vi "X682 Camera Calibration Tester Program Ver1.0.0.0.vi"() -> ()   [LabVIEW 2017]
uses:
  Thorlabs.MotionControl.Controls.dll
  Ctrls/MainStep.ctl
  Ctrls/AllControls.ctl
  <vilib>/Utility/miscctls.llb/LVRowAndColumnTypeDef.ctl
  ComVIS/Files/Ini/WriteIniFiles_ByVarient.vi
  Thorlabs.MotionControl.IntegratedStepperMotorsCLI.dll
panel:
  in  "LongTravelStageControl":refnum<k24>(container)
  in  "Recipe":string(combo)
  in  "MES Status":bool
  in  "maintenance":bool
  in  "mode":enum32{"Production mode", "Engineering mode"}(tab)
  out "Fail resume":bool caption="TotalResult"
  out "Table":string[][](table)
  out "LogInfo":string caption="Log"
  in  "AlarmData":i32(listbox)=-1
  out "Device state":bool caption="TotalResult"
  out "CT":dbl format="%#_3f"
  in  "ProductID:":string
  in  "TestInfo":T1 {"Yield" format="%#_g%"}
  out "MES_Status":string
  out "TestMode":string
  in  "Stop":bool
  in  "Start":bool
  in  "Exit":bool
  in  "Login":bool
  out "Login_status":string="Operator:Operator"
  out "OpenStatus":string
  in  "error in (no error)":errorcluster caption="错误输入（无错误）"
  # "Dyson X682 Camera Calibration Tester"
  # "Waiting Barcode scanning"
types:
  T1 = cluster{"Total":i32, "OK":i32, "NG":i32, "Yield":dbl}
  T2 = typedef "MainStep.ctl" = enum16{"Initialize", "ReadAllFiles", "ResetHardware", "Run", "Exit"}
  T3 = typedef "AllControls.ctl" = cluster{"MainVI":refnum<vi>, "AlarmInfo":refnum<vi>, "Log":refnum<vi>, "Current CT":refnum<vi>, "ProductID":refnum<vi>, "Device state":refnum<vi>, "MES":refnum<vi>, "mode":refnum<vi>, "TestInfo":refnum<vi>, "SubPnl":refnum<vi>, "Table":refnum<vi>, "MES bool":refnum<vi>, "TestMode":refnum<vi>, "Recipe":refnum<vi>, "Fail resume":refnum<vi>, "LogIn":refnum<vi>, "Start":refnum<vi>, "Maintenance":refnum<vi>, "Stop":refnum<vi>, "Exit":refnum<vi>}
  T4 = enum32{"Invalid", "Standard", "Closed", "Hidden", "Minimized", "Maximized"}
  T5 = enum16{"Ini", "Standby", "Running", "Engineering"}
  T6 = typedef "LVRowAndColumnTypeDef.ctl" = cluster{"Row":i32, "Column":i32}
  T7 = enum32{"invalid app kind", "Development System", "Run Time System", "Student Edition", "Embedded LabVIEW", "Evaluation", "Custom"}
  T8 = typedef "amc_Message Queue.ctl" = refnum<queue>
  T9 = typedef "HD Config.ctl" = cluster{" PC":cluster{"PC Address":u8[], "PC Port":i32}, "FCO":cluster{"COM":refnum<visa-resource-name>, "Baudrate":u32}, "DC Power ":cluster{"COM":refnum<visa-resource-name>, "Baudrate":u32}, "PW3336":cluster{"COM":refnum<visa-resource-name>, "Baudrate":u32}, "Lefoo":cluster{"COM":refnum<visa-resource-name>, "Baudrate":u32}, "Tempt&Hum":cluster{"COM":refnum<visa-resource-name>, "Baudrate":u32}, "DIPC":cluster{"COM":refnum<visa-resource-name>}, "Daemon":cluster{"IP Address":string, "Port":u16, "Retry":u16}, "NFC_Cmd":cluster{"COM":refnum<visa-resource-name>, "Baudrate":u32}, "Fail_resume_mode":bool, "GRR":bool, "NFC _Serial":cluster{"COM":refnum<visa-resource-name>, "Baudrate":u32}}
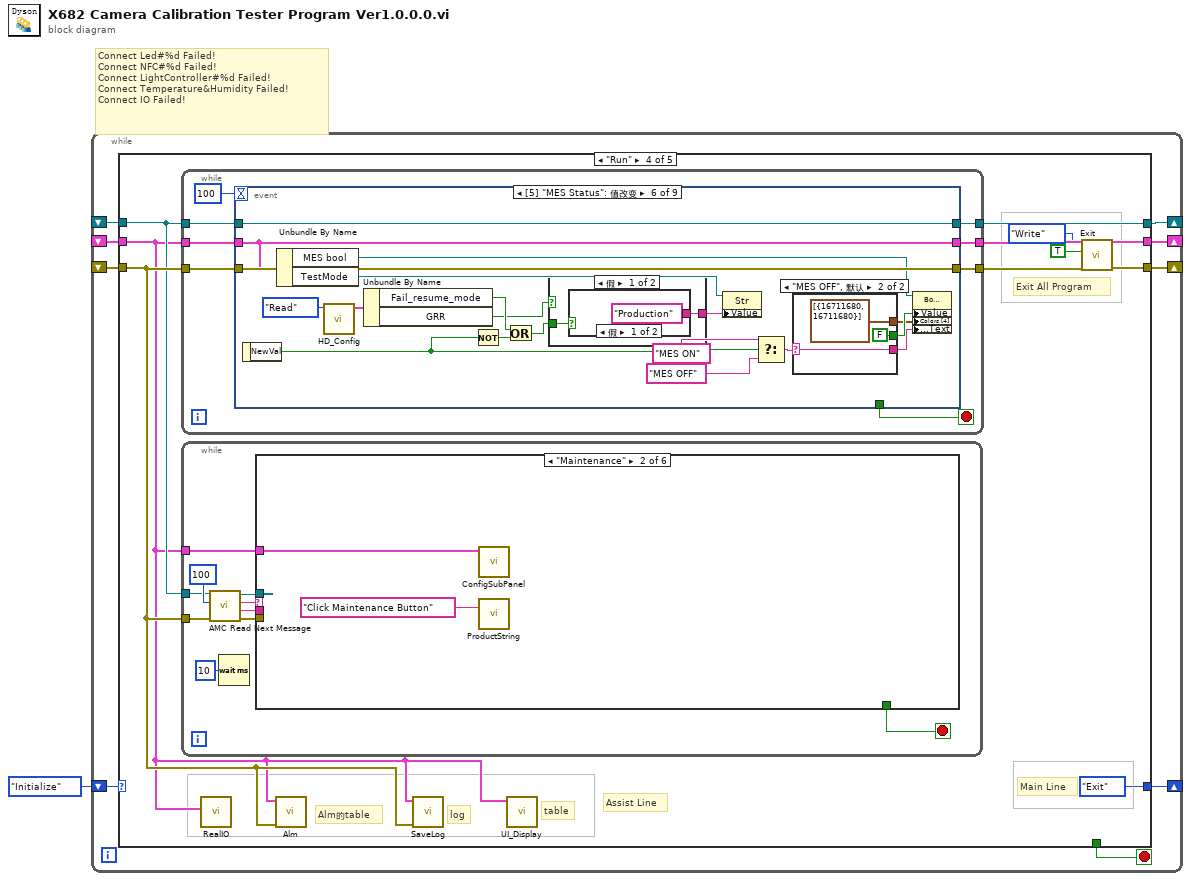
[diagram p0: block diagram]
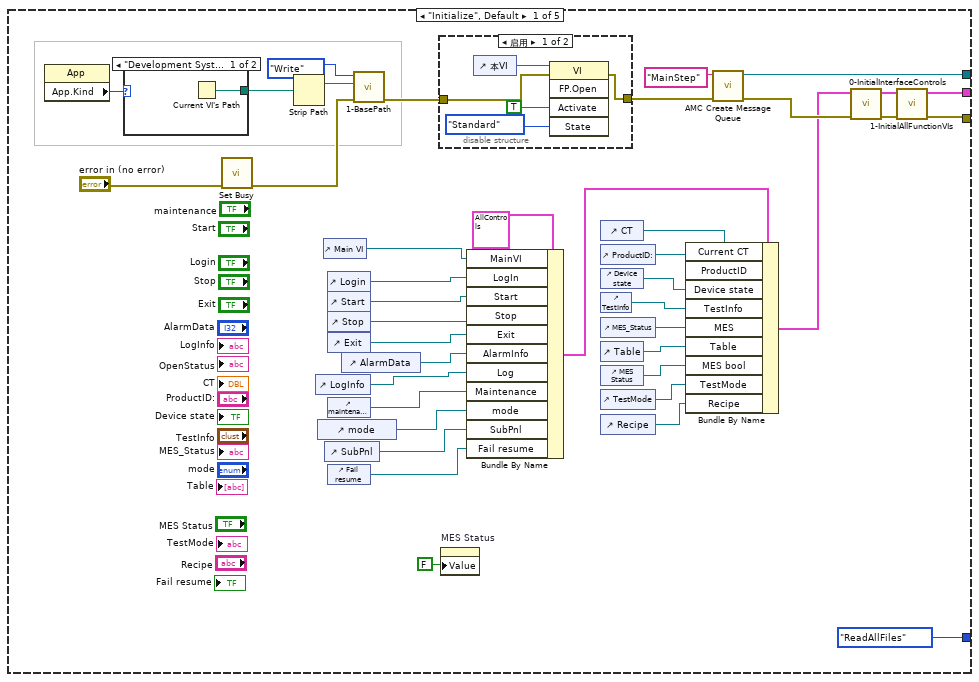
[diagram p2: hidden frame]
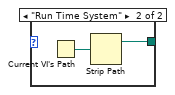
[diagram p4: hidden frame]
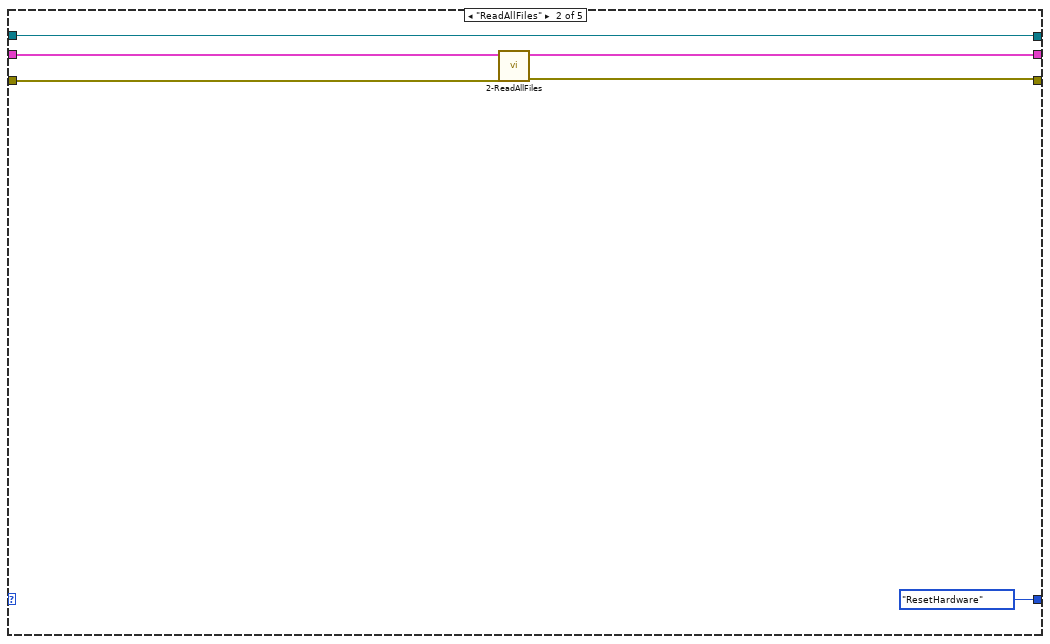
[diagram p5: hidden frame]
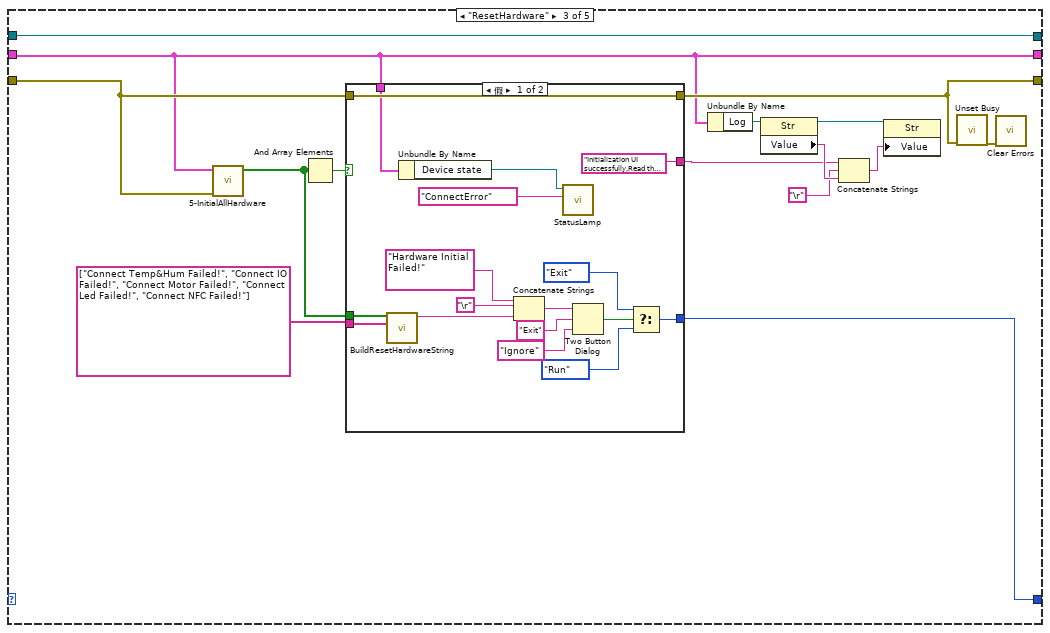
[diagram p6: hidden frame]
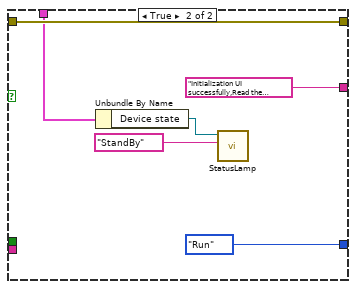
[diagram p7: hidden frame]
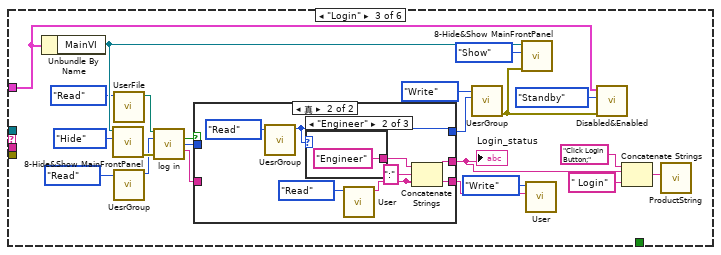
[diagram p9: hidden frame]
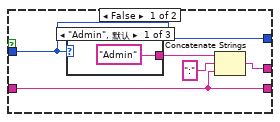
[diagram p10: hidden frame]
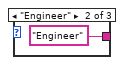
[diagram p11: hidden frame]
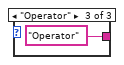
[diagram p12: hidden frame]
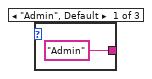
[diagram p13: hidden frame]
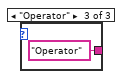
[diagram p14: hidden frame]
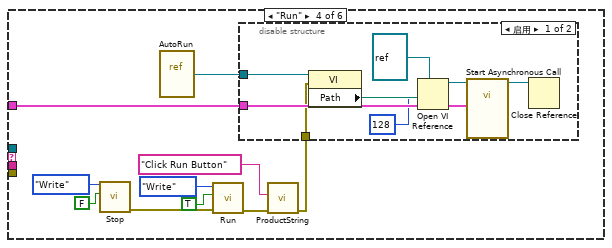
[diagram p15: hidden frame]
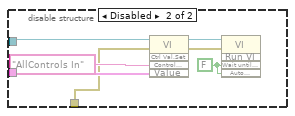
[diagram p16: hidden frame]
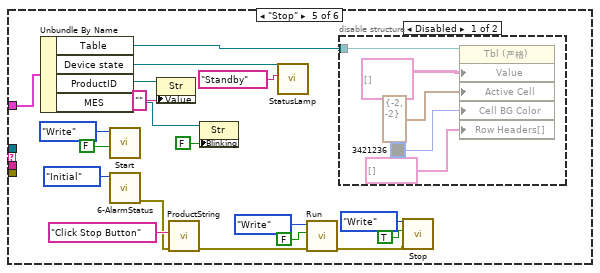
[diagram p17: hidden frame]
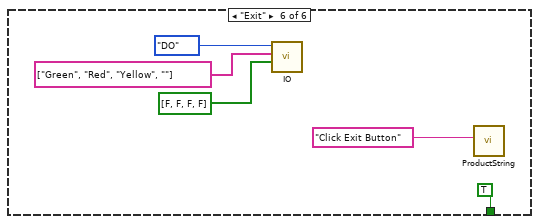
[diagram p19: hidden frame]
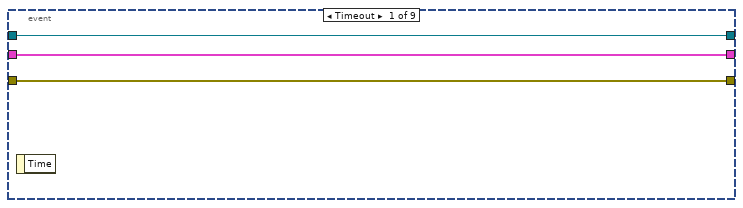
[diagram p20: hidden frame]
diagram:
  # "Connect Led#%d Failed!\nConnect NFC#%d Failed!\nConnect LightController#%d Failed!\nConnect Temperature&Humidity Failed!\nConnect IO Failed!"
  n1 = while {
    shift-right: [w9] -> _
    shift-left: MainStep."Initialize" -> [w10]
    shift-right: [w7] -> _
    shift-left: _ -> [w2]
    shift-right: [w5] -> _
    shift-left: _ -> [w3]
    shift-right: [w6] -> _
    shift-left: _ -> [w4]
    stop <- w8 stop-if-true
    n2 = case shown="\"Run\"" w10 {
      tunnel: [MainStep."ReadAllFiles" MainStep."ResetHardware" w80 MainStep."Exit" MainStep."Exit"] -> w9
      tunnel: [_ _ _ _ TRUE] -> w8
      tunnel: [w37 w60 w76 w107 w347] -> w7
      tunnel: [w45 w64 w79 w112 _] -> w6
      tunnel: [w38 w62 w74 w111 w345] -> w5
      tunnel: w4 -> [_ w64 w79 w105 w348]
      tunnel: w3 -> [_ w63 w74 w104 w345]
      tunnel: w2 -> [_ w61 w77 w106 w346]
      frame "Initialize", Default {
        n3 = property class="App"() -> ("App.Kind"=w49:T7)  [unwired: 2 in, 2 out]
        n4 = case shown="\"Development System\", 默认" w49 {
          tunnel: [w57 w58] -> w48
          frame "Development System", Default {
            n5 = Current VI's Path() -> (path=w57:path)
          }
          frame "Run Time System" {
            n6 = Current VI's Path() -> (path=w59:path)
            n7 = Strip Path(path=w59) -> (stripped path=w58:path)  [unwired: 1 out]
          }
        }
        n8 = call <vilib>:"Set Busy.vi"("error in (no error)"="error in (no error)") -> ("error out"=w17:errorcluster)  [unwired: 9 in, 1 out]
        n9 = Strip Path(path=w48) -> (stripped path=w18:path)  [unwired: 1 out]
        n10 = control-ref of="LogInfo"() -> (w42:refnum<vi>)
        n11 = control-ref of="mode"() -> (w24:refnum<vi>)
        n12 = control-ref of="Main VI"() -> (w35:refnum<vi>)
        n13 = control-ref of="SubPnl"() -> (w22:refnum<vi>)
        n14 = control-ref of="Login"() -> (w25:refnum<vi>)
        n15 = control-ref of="Start"() -> (w26:refnum<vi>)
        n16 = control-ref of="Stop"() -> (w27:refnum<vi>)
        n17 = control-ref of="Exit"() -> (w28:refnum<vi>)
        n18 = control-ref of="maintenance"() -> (w23:refnum<vi>)
        n19 = control-ref of="Fail resume"() -> (w12:refnum<vi>)
        n20 = control-ref of="AlarmData"() -> (w43:refnum<vi>)
        n21 = call "1-BasePath.vi"("error in (no error)"=w17, "Path In"=w18, "Step"=enum16{"Initial", "Write", "Read"}."Write") -> ("error out"=w16:errorcluster)  [unwired: 7 in, 1 out]
        n22 = disable-structure shown="启用" {
          disable-tunnel: w16 -> [w53 w56]
          disable-tunnel: [w51 w56] -> w46
          frame Enabled {
            n23 = control-ref of="本VI"() -> (w55:refnum<vi>)
            n24 = invoke class="VI" method="FP.Open"(reference=w55, error in=w53, "Activate"=TRUE ("激活？"), "State"=T4."Standard" ("状态")) -> (error out=w51:errorcluster)  [unwired: 1 in, 4 out]
          }
          frame Disabled {
          }
        }
        n25 = property on="MES Status" class="Bool (严格)"("Value"=FALSE ("MES Status")) -> ()  [unwired: 2 in, 2 out]
        n26 = Bundle By Name(cluster=T3 {"MainVI"=refnum, "AlarmInfo"=refnum, "Log"=refnum, "Current CT"=refnum, "ProductID"=refnum, "Device state"=refnum, "MES"=refnum, "mode"=refnum, "TestInfo"=refnum, "SubPnl"=refnum, "Table"=refnum, "MES bool"=refnum, "TestMode"=refnum, "Recipe"=refnum, "Fail resume"=refnum, "LogIn"=refnum, "Start"=refnum, "Maintenance"=refnum, "Stop"=refnum, "Exit"=refnum}, "MainVI"=w35, "LogIn"=w25, "Start"=w26, "Stop"=w27, "Exit"=w28, "AlarmInfo"=w43, "Log"=w42, "Maintenance"=w23, "mode"=w24, "SubPnl"=w22, "Fail resume"=w12) -> (w34:T3)
        n27 = control-ref of="CT"() -> (w31:refnum<vi>)
        n28 = control-ref of="ProductID:"() -> (w32:refnum<vi>)
        n29 = control-ref of="Device state"() -> (w33:refnum<vi>)
        n30 = control-ref of="TestInfo"() -> (w30:refnum<vi>)
        n31 = control-ref of="MES_Status"() -> (w29:refnum<vi>)
        n32 = control-ref of="Table"() -> (w20:refnum<vi>)
        n33 = control-ref of="MES Status"() -> (w15:refnum<vi>)
        n34 = control-ref of="TestMode"() -> (w14:refnum<vi>)
        n35 = control-ref of="Recipe"() -> (w13:refnum<vi>)
        n36 = Bundle By Name(cluster=w34, "Current CT"=w31, "ProductID"=w32, "Device state"=w33, "TestInfo"=w30, "MES"=w29, "Table"=w20, "MES bool"=w15, "TestMode"=w14, "Recipe"=w13) -> (w21:T3)
        n37 = call "AMC Create Message Queue.vi"("error in (no error)"=w46, "Message Queue Name"="MainStep" ("Message queue name (unnamed)")) -> ("error out"=w41:errorcluster, "Message Queue out"=w45:T8)  [unwired: 3 in, 5 out]
        n38 = call "0-InitialInterfaceControls.vi"("error in (no error)"=w41, "AllControls IN"=w21) -> ("error out"=w40:errorcluster, "AllControls Out"=w39:T3)  [unwired: 8 in]
        n39 = call "1-InitialAllFunctionVIs.vi"("error in (no error)"=w40, "AllControls IN"=w39) -> ("error out"=w37:errorcluster, "AllControls Out"=w38:T3)  [unwired: 8 in]
      }
      frame "ReadAllFiles" {
        n40 = call "2-ReadAllFiles.vi"("error in (no error)"=w61, "AllControls IN"=w63) -> ("error out"=w60:errorcluster, "AllControls Out"=w62:T3)  [unwired: 8 in]
      }
      frame "ResetHardware" {
        n41 = call "5-InitialAllHardware.vi"("error in (no error)"=w77, "AllControls IN"=w74) -> ("InitalResult"=w78:bool[])  [unwired: 9 in]
        n42 = And Array Elements(Boolean array=w78) -> (logical AND=w66:bool)
        n43 = case shown="假" w66 {
          tunnel: [w88 MainStep."Run"] -> w80
          tunnel: w77 -> [w97 w102]
          tunnel: string[] ["Connect Temp&Hum Failed!", "Connect IO Failed!", "Connect Motor Failed!", "Connect Led Failed!", "Connect NFC Failed!"] -> [w86 _]
          tunnel: w78 -> [w87 _]
          tunnel: [w97 w102] -> w76
          tunnel: ["Initialization UI successfully,Read the configuration parameter successfully,Initialize hardware failure" ("值") "Initialization UI successfully,Read the configuration parameter successfully,Initialize hardware successfully" ("值")] -> w70
          tunnel: w74 -> [w81 w100]
          frame False {
            n44 = call "BuildResetHardwareString.vi"("String"=w86, "Error"=w87) -> ("DataOut"=w85:string)  [unwired: 9 in]
            n45 = Unbundle By Name(w81) -> ("Device state"=w82:refnum<vi>)
            n46 = Concatenate Strings("Hardware Initial Failed!" ("caption"), "\r", w85) -> (w95:string)
            n47 = call "StatusLamp.vi"("State"="ConnectError", "Boolean输入"=w82) -> ()  [unwired: 9 in, 1 out]
            n48 = Two Button Dialog(message=w95, 1:"Ignore" ("F按钮名称（“取消”）"), 2:"Exit" ("T按钮名称（“确定”）")) -> (T button?=w91:bool)
            n49 = Select(t=MainStep."Exit", s=w91, f=MainStep."Run") -> (s? t:f=w88:T2)
          }
          frame True {
            n50 = Unbundle By Name(w100) -> ("Device state"=w98:refnum<vi>)
            n51 = call "StatusLamp.vi"("State"="StandBy", "Boolean输入"=w98) -> ()  [unwired: 9 in, 1 out]
          }
        }
        n52 = Unbundle By Name(w74) -> ("Log"=w71:refnum<vi>)
        n53 = property class="Str"(reference=w71) -> (reference out=w69:refnum<vi>, "Value"=w73:string)  [unwired: 1 in, 1 out]
        n54 = Concatenate Strings(w70, "\r", w73) -> (w68:string)
        n55 = property class="Str"(reference=w69, "Value"=w68) -> ()  [unwired: 1 in, 2 out]
        n56 = call <vilib>:"Unset Busy.vi"("error in (no error)"=w76) -> ("error out"=w75:errorcluster)  [unwired: 10 in]
        n57 = call <vilib>:"Clear Errors.vi"("error in (no error)"=w75) -> ()  [unwired: 5 in, 2 out]
      }
      frame "Run" {
        # "Alm的table"
        # "log"
        # "table"
        # "Exit All Program"
        # "Assist Line"
        # "Main Line"
        n58 = while {
          tunnel: w105 -> [w227]
          tunnel: w104 -> [w226]
          tunnel: w106 -> [w225]
          tunnel: [w224] -> w112
          tunnel: [w223] -> w111
          tunnel: [w222] -> w108
          stop <- w221 stop-if-true
          n59 = event shown="[5] \"MES Status\": 值改变" {
            selector: _ -> [_ _ _ _ _ _ _ _ _]
            dyn-events: _ -> [_ _ _ _ _ _ _ _ _]
            timeout: 100 -> [_ _ _ _ _ _ _ _ _]
            tunnel: w227 -> [w230 w238 w263 w269 w281 w306 w320 w329 w336]
            tunnel: w226 -> [w229 w233 w261 w268 w279 w304 w318 w331 w341]
            tunnel: w225 -> [w228 w237 w262 w271 w280 w305 w319 w328 w337]
            tunnel: [w230 w238 w263 w269 w281 w306 w320 w329 w336] -> w224
            tunnel: [w229 w233 w261 w268 w279 w304 w318 w331 w341] -> w223
            tunnel: [w228 w237 w262 w271 w280 w305 w319 w328 w337] -> w222
            tunnel: [_ _ _ _ _ _ _ w327 w340] -> w221
            event Timeout {
              n60 = event-data() -> ()  [unwired: 1 in, 1 out]
            }
            event "Recipe": Value Change {
              n61 = event-data() -> ("OldVal"=w236:string, "NewVal"=w234:string)  [unwired: 1 in]
              n62 = Not Equal?(x=w236, y=w234) -> (x != y?=w235:bool)
              n63 = call "Run.vi"("Step"=enum16{"Initial", "Write", "Read"}."Read") -> ("Run Out"=w231:bool)  [unwired: 9 in, 1 out]
              n64 = case shown="假" w231 {
                tunnel: w235 -> [w241 _]
                tunnel: w234 -> [w240 _]
                tunnel: w233 -> [w239 _]
                frame False {
                  n65 = case shown="真" w241 {
                    tunnel: w240 -> [_ w255]
                    tunnel: w239 -> [_ w243]
                    frame False {
                    }
                    frame True {
                      w256 = cluster{"Recipe":string} {"Recipe"=""}  # Recipe
                      n66 = call "1-BasePath.vi"("Step"=enum16{"Initial", "Write", "Read"}."Read") -> ("Path Out"=w257:path)  [unwired: 9 in, 1 out]
                      n67 = call "ReadConfigandSetting.vi"("Recipe"=w255, "Path Out"=w257) -> ("TableData"=w244:string[][])  [unwired: 7 in, 2 out]
                      n68 = Bundle By Name(cluster=w256, "Recipe"=w255) -> (w254:cluster{"Recipe":string})
                      n69 = Build Path(base path=w257, name or relative path="data\\Recipe.ini") -> (appended path=w259:path)
                      n70 = Unbundle By Name(w243) -> ("Table"=w242:refnum<vi>)
                      n71 = call-poly "Read&WriteFile.vi"("Variant"=w254, "path"=w259) -> ()  [unwired: 9 in, 1 out]
                      n72 = Delete From Array(array=w244, length=1 ("长度"), index (row)=0 ("索引 (行)")) -> (deleted portion=w252:string[][], array with subset deleted=w250:string[][])  [unwired: 1 in]
                      n73 = call "Select_UUT_Table.vi"("all Title"=w252, "all Table"=w250) -> ("Title"=w251:string[], "Table"=w253:string[][])  [unwired: 8 in]
                      n74 = property class="Tbl (严格)"(reference=w242, "Value"=w253, "Column Headers[]"=w251, "Active Cell"=T6 {"Row"=-2, "Column"=-2} ("活动单元格:活动单元格"), "Cell BG Color"=u32 3421236, "Row Headers[]"=string[] [] ("Row Header Strings[]")) -> ()  [unwired: 1 in, 2 out]
                    }
                  }
                }
                frame True {
                }
              }
            }
            event "Login": Value Change {
              n75 = event-data() -> ("NewVal"=w264:bool)  [unwired: 1 in]
              n76 = case shown="真" w264 {
                tunnel: w263 -> [w267 _]
                tunnel: w262 -> [w266 _]
                frame True {
                  n77 = call "AMC Send Local Message.vi"("error in (no error)"=w266, "Message Name"="Login", "Message Queue in"=w267) -> ()  [unwired: 7 in, 2 out]
                }
                frame False {
                }
              }
            }
            event "maintenance": Value Change {
              n78 = event-data() -> ("NewVal"=w272:bool)  [unwired: 1 in]
              n79 = Unbundle By Name(w268) -> ("mode"=w270:refnum<vi>)
              n80 = case shown="真" w272 {
                tunnel: w270 -> [w278 _]
                tunnel: w269 -> [w275 _]
                tunnel: w268 -> [w274 _]
                frame True {
                  n81 = call "AMC Send Local Message.vi"("Message Name"="Maintenance", "Message Queue in"=w275) -> ()  [unwired: 8 in, 2 out]
                  n82 = property class="TabCtl (严格)"(reference=w278, "Value"=enum32{"Production mode", "Engineering mode"}."Engineering mode" ("值")) -> ()  [unwired: 1 in, 2 out]
                  n83 = call "Disabled&Enabled.vi"("Mode in"=T5."Engineering", "AllControls In"=w274) -> ()  [unwired: 9 in, 1 out]
                }
                frame False {
                }
              }
            }
            event "Start": Value Change {
              n84 = event-data() -> ("NewVal"=w282:bool)  [unwired: 1 in]
              n85 = case shown="真" w282 {
                tunnel: w281 -> [w287 _]
                tunnel: w280 -> [w286 _]
                tunnel: w279 -> [w283 _]
                frame True {
                  n86 = call "AMC Send Local Message.vi"("error in (no error)"=w286, "Message Name"="Run", "Message Queue in"=w287) -> ()  [unwired: 7 in, 2 out]
                  n87 = call "Disabled&Enabled.vi"("Mode in"=T5."Running", "AllControls In"=w283) -> ()  [unwired: 9 in, 1 out]
                }
                frame False {
                }
              }
            }
            event "MES Status": Value Change {
              n88 = event-data() -> ("NewVal"=w289:bool)  [unwired: 1 in]
              n89 = Unbundle By Name(w304) -> ("MES bool"=w297:refnum<vi>, "TestMode"=w288:refnum<vi>)
              n90 = call "HD_Config.vi"("Step"=enum16{"Initial", "Write", "Read"}."Read") -> ("HD Config out"=w296:T9)  [unwired: 9 in, 1 out]
              n91 = Unbundle By Name(w296) -> ("Fail_resume_mode"=w293:bool, "GRR"=w291:bool)
              n92 = Not(x=w289) -> (.not. x?=w295:bool)
              n93 = Or(x=w293, y=w295) -> (x .or. y?=w294:bool)
              n94 = case shown="假" w291 {
                tunnel: w294 -> [w308 _]
                tunnel: [w307 "GRR"] -> w292
                frame False {
                  n95 = case shown="假" w308 {
                    tunnel: ["Production" "Engineering"] -> w307
                    frame False {
                    }
                    frame True {
                    }
                  }
                }
                frame True {
                }
              }
              n96 = property class="Str"(reference=w288, "Value"=w292) -> ()  [unwired: 1 in, 2 out]
              n97 = Select(t="MES ON", s=w289, f="MES OFF") -> (s? t:f=w298:string)
              n98 = case shown="\"MES OFF\", 默认" w298 {
                selector: w298 -> [w312 w315]
                tunnel: [TRUE FALSE] -> w300
                tunnel: [w312 w315] -> w301
                tunnel: [cluster{u32, u32}[] [{6618880, 6618880}] cluster{u32, u32}[] [{16711680, 16711680}]] -> w299
                frame "MES ON" {
                }
                frame "MES OFF", Default {
                }
              }
              n99 = property on="属性节点" class="Bool (严格)"(reference=w297, "Value"=w300, "Colors [4]"=w299, "BoolText.Text"=w301) -> ()  [unwired: 1 in, 2 out]
            }
            event "Stop": Value Change {
              n100 = event-data() -> ("NewVal"=w321:bool)  [unwired: 1 in]
              n101 = case shown="真" w321 {
                tunnel: w320 -> [w326 _]
                tunnel: w319 -> [w325 _]
                tunnel: w318 -> [w322 _]
                frame True {
                  n102 = call "AMC Send Local Message.vi"("error in (no error)"=w325, "Message Name"="Stop", "Message Queue in"=w326) -> ()  [unwired: 7 in, 2 out]
                  n103 = call "Disabled&Enabled.vi"("Mode in"=T5."Standby", "AllControls In"=w322) -> ()  [unwired: 9 in, 1 out]
                }
                frame False {
                }
              }
            }
            event "Exit": Value Change {
              n104 = event-data() -> ("NewVal"=w330:bool)  [unwired: 1 in]
              n105 = case shown="真" w330 {
                tunnel: w329 -> [_ w335]
                tunnel: w328 -> [_ w334]
                tunnel: [_ TRUE] -> w327
                frame False {
                }
                frame True {
                  n106 = call "AMC Send Local Message.vi"("error in (no error)"=w334, "Message Name"="Exit", "Message Queue in"=w335) -> ()  [unwired: 7 in, 2 out]
                }
              }
            }
            event Panel Close? {
              n107 = event-data() -> ()  [unwired: 1 in, 1 out]
              n108 = Two Button Dialog(message="Are you sure to Exit system?") -> (T button?=w339:bool)  [unwired: 2 in]
              n109 = case shown="假" w339 {
                selector: w339 -> [w343 w344]
                tunnel: [w343 w344] -> w340
                frame False {
                }
                frame True {
                }
              }
              n110 = Not(x=w340) -> (.not. x?=w342:bool)
              n111 = event-data("Discard?"=w342) -> ()  [unwired: 1 in, 1 out]
            }
          }
        }
        n112 = while {
          tunnel: w104 -> [w123]
          tunnel: w106 -> [w120]
          tunnel: w105 -> [w117]
          stop <- w114 stop-if-true
          n113 = call "AMC Read Next Message.vi"("error in (no error)"=w120, "timeout (1ms)"=100 ("Timeout"), "Message Queue in"=w117) -> ("error out"=w119:errorcluster, "Message Value"=w115:string, "Message Name"=w118:string, "Message Queue out"=w116:T8)  [unwired: 1 in, 4 out]
          n114 = Wait (ms)(milliseconds to wait=u32 10 ("毫秒倍数")) -> ()  [unwired: 1 out]
          n115 = case shown="\"Maintenance\"" w118 {
            tunnel: w123 -> [_ w125 w133 w168 w208 _]
            tunnel: w119 -> [_ _ _ _ _ _]
            tunnel: [_ _ _ _ _ TRUE] -> w114
            tunnel: w116 -> [_ _ _ _ _ _]
            tunnel: w115 -> [_ _ _ _ _ _]
            frame "Null", Default {
            }
            frame "Maintenance" {
              n116 = call "ConfigSubPanel.vi"("AllControls"=w125) -> ()  [unwired: 11 in]
              n117 = call "ProductString.vi"("String"="Click Maintenance Button" ("值")) -> ()  [unwired: 10 in, 1 out]
            }
            frame "Login" {
              n118 = Unbundle By Name(w133) -> ("MainVI"=w146:refnum<vi>)
              n119 = call "8-Hide&Show MainFrontPanel.vi"("Hide&Show"=enum16{"Hide", "Show"}."Hide", "This VI"=w146) -> ("error out"=w144:errorcluster)  [unwired: 9 in]
              n120 = call "UserFile.vi"("Step"=enum16{"Initial", "Write", "Read"}."Read") -> ("UserPath out"=w143:path)  [unwired: 9 in, 1 out]
              n121 = call "UesrGroup.vi"("Step"=enum16{"Initial", "Write", "Read"}."Read") -> ("User group out"=w126:enum16{"Operator", "Engineer", "Admin"})  [unwired: 9 in, 1 out]
              n122 = call "log in.vi"("路径"=w143, "UserGroups in"=w126, "error in (no error)"=w144) -> ("Giveup?"=w141:bool, "UserGroups"=w140:enum16{"Operator", "Engineer", "Admin"}, "User"=w139:string)  [unwired: 8 in, 2 out]
              n123 = case shown="真" w141 {
                tunnel: [w149 w156] -> w135
                tunnel: [w150 w160] -> w129
                tunnel: [w148 w158] -> w137
                tunnel: w140 -> [w148 _]
                tunnel: w139 -> [w149 _]
                frame False {
                  n124 = case shown="\"Admin\", 默认" w148 {
                    tunnel: ["Admin" "Engineer" "Operator"] -> w152
                    frame "Admin", Default {
                    }
                    frame "Engineer" {
                    }
                    frame "Operator" {
                    }
                  }
                  n125 = Concatenate Strings(w152, ":" ("字符串"), w149) -> (w150:string)
                }
                frame True {
                  n126 = call "UesrGroup.vi"("Step"=enum16{"Initial", "Write", "Read"}."Read") -> ("User group out"=w158:enum16{"Operator", "Engineer", "Admin"})  [unwired: 9 in, 1 out]
                  n127 = case shown="\"Engineer\"" w158 {
                    tunnel: ["Admin" "Engineer" "Operator"] -> w162
                    frame "Admin", Default {
                    }
                    frame "Engineer" {
                    }
                    frame "Operator" {
                    }
                  }
                  n128 = call "User.vi"("Step"=enum16{"Initial", "Write", "Read"}."Read") -> ("User out"=w156:string)  [unwired: 9 in, 1 out]
                  n129 = Concatenate Strings(w162, ":" ("字符串"), w156) -> (w160:string)
                }
              }
              "Login_status" <- w129
              n130 = call "UesrGroup.vi"("User group in"=w137, "Step"=enum16{"Initial", "Write", "Read"}."Write") -> ("错误输出"=w132:errorcluster)  [unwired: 8 in, 1 out]
              n131 = call "8-Hide&Show MainFrontPanel.vi"("error in (no error)"=w132, "Hide&Show"=enum16{"Hide", "Show"}."Show", "This VI"=w146) -> ()  [unwired: 8 in, 1 out]
              n132 = call "User.vi"("User in"=w135, "Step"=enum16{"Initial", "Write", "Read"}."Write") -> ()  [unwired: 8 in, 2 out]
              n133 = call "Disabled&Enabled.vi"("error in (no error)"=w132, "Mode in"=T5."Standby", "AllControls In"=w133) -> ()  [unwired: 8 in, 1 out]
              n134 = Concatenate Strings("Click Login Button;" ("String"), w129, " Login" ("字符串")) -> (w130:string)
              n135 = call "ProductString.vi"("String"=w130) -> ()  [unwired: 10 in, 1 out]
            }
            frame "Run" {
              n136 = call "Stop.vi"("Stop In"=FALSE ("AutoStopping In"), "Step"=enum16{"Initial", "Write", "Read"}."Write") -> ("error out"=w174:errorcluster)  [unwired: 8 in, 1 out]
              n137 = vi-ref "AutoRun.vi"() -> (w166:refnum<vi>)
              n138 = call "Run.vi"("error in (no error)"=w174, "Run In"=TRUE ("AutoRun In"), "Step"=enum16{"Initial", "Write", "Read"}."Write") -> ("error out"=w169:errorcluster)  [unwired: 7 in, 1 out]
              n139 = call "ProductString.vi"("error"=w169, "String"="Click Run Button" ("值")) -> ("error  out"=w167:errorcluster)  [unwired: 9 in]
              n140 = disable-structure shown="启用" {
                disable-tunnel: w168 -> [w180 w186]
                disable-tunnel: w167 -> [w178 w184]
                disable-tunnel: w166 -> [w177 w185]
                frame Enabled {
                  n141 = property class="VI"(reference=w177, error in=w178) -> ("Path"=w183:path)  [unwired: 2 out]
                  n142 = Open VI Reference(type specifier VI Refnum (for type only)=refnum<vi> refnum ("application reference (local)"), vi path=w183, options=128) -> (vi reference=w181:refnum<vi>)  [unwired: 3 in, 1 out]
                  n143 = call-by-ref "Start Asynchronous Call"(reference=w181, "AllControls In"=w180) -> (reference out=w179:refnum<vi>)  [unwired: 12 in, 1 out]
                  n144 = Close Reference(reference=w179) -> ()  [unwired: 1 in, 1 out]
                }
                frame Disabled {
                  w187 = FALSE ("Wait Until Done")
                  n145 = invoke class="VI" method="Ctrl Val.Set"(reference=w185, error in=w184, "Control Name"="AllControls In", "Value"=w186) -> (reference out=w189:refnum<vi>, error out=w190:errorcluster)  [unwired: 1 in, 3 out]
                  n146 = invoke class="VI" method="Run VI"(reference=w189, error in=w190, "Wait until done"=w187, "Auto Dispose Ref"=w187) -> ()  [unwired: 1 in, 5 out]
                }
              }
            }
            frame "Stop" {
              n147 = Unbundle By Name(w208) -> ("Table"=w197:refnum<vi>, "Device state"=w205:refnum<vi>, "ProductID"=w207:refnum<vi>, "MES"=w192:refnum<vi>)
              n148 = call "Start.vi"("Start In"=FALSE, "Step"=enum16{"Initial", "Write", "Read"}."Write") -> ()  [unwired: 8 in, 2 out]
              n149 = call "6-AlarmStatus.vi"("Step"=enum16{"Initial", "Write", "Read"}."Initial") -> ("error out"=w193:errorcluster)  [unwired: 9 in, 1 out]
              n150 = property class="Str"(reference=w207, "Value"="") -> ()  [unwired: 1 in, 2 out]
              n151 = call "ProductString.vi"("error"=w193, "String"="Click Stop Button" ("值")) -> ("error  out"=w198:errorcluster)  [unwired: 9 in]
              n152 = property class="Str"(reference=w192, "Blinking"=FALSE ("闪烁")) -> ()  [unwired: 1 in, 2 out]
              n153 = call "StatusLamp.vi"("State"="Standby", "Boolean输入"=w205) -> ()  [unwired: 9 in, 1 out]
              n154 = call "Run.vi"("error in (no error)"=w198, "Run In"=FALSE ("AutoRun In"), "Step"=enum16{"Initial", "Write", "Read"}."Write") -> ("error out"=w203:errorcluster)  [unwired: 7 in, 1 out]
              n155 = disable-structure shown="Disabled" {
                disable-tunnel: w197 -> [w211 _]
                frame Disabled {
                  n156 = property class="Tbl (严格)"(reference=w211, "Value"=string[][] [] ("值"), "Active Cell"=T6 {"Row"=-2, "Column"=-2} ("活动单元格:活动单元格"), "Cell BG Color"=u32 3421236, "Row Headers[]"=string[] [] ("Row Header Strings[]")) -> ()  [unwired: 1 in, 2 out]
                }
                frame Enabled {
                }
              }
              n157 = call "Stop.vi"("error in (no error)"=w203, "Stop In"=TRUE ("AutoStopping In"), "Step"=enum16{"Initial", "Write", "Read"}."Write") -> ()  [unwired: 7 in, 2 out]
            }
            frame "Exit" {
              n158 = call "IO.vi"("DO DATA"=bool[] [FALSE, FALSE, FALSE, FALSE], "IO Name"=string[] ["Green", "Red", "Yellow", ""], "IO?"=enum16{"DI", "DO"}."DO") -> ()  [unwired: 7 in, 2 out]
              n159 = call "ProductString.vi"("String"="Click Exit Button" ("值")) -> ()  [unwired: 10 in, 1 out]
            }
          }
        }
        n160 = call "RealIO.vi"("AllControls Out"=w104) -> ()  [unwired: 11 in]
        n161 = call "Alm.vi"("error in (no error)"=w106, "AllControls Out"=w104) -> ()  [unwired: 10 in]
        n162 = call "SaveLog.vi"("错误输入（无错误）"=w106, "AllControls In"=w104) -> ()  [unwired: 9 in, 1 out]
        n163 = call "UI_Display.vi"("AllControls In"=w104) -> ()  [unwired: 11 in]
        n164 = call "Exit.vi"("error in (no error)"=w108, "Exit In"=TRUE, "Step"=enum16{"Initial", "Write", "Read"}."Write" ("step")) -> ("error out"=w107:errorcluster)  [unwired: 7 in, 1 out]
      }
      frame "Exit" {
        n165 = disable-structure shown="Disabled" {
          frame Disabled {
            n166 = property class="LongTravelStageControl"(reference="LongTravelStageControl", "SerialNumber"="") -> (reference out=w353:refnum<k24>, error out=w355:errorcluster)  [unwired: 1 in]
            n167 = invoke class="LongTravelStageControl" method="CreateDevice"(reference=w353, error in=w355) -> (reference out=w354:refnum<k24>, error out=w356:errorcluster)  [unwired: 1 in, 1 out]
            n168 = property class="LongTravelStageControl"(reference=w354, error in=w356) -> (error out=w359:errorcluster, "Device"=w358:refnum<k24>)  [unwired: 1 out]
            n169 = invoke class="IntegratedStepperMotor" method="Home"(reference=w358, error in=w359, "waitTimeout"=200000) -> ()  [unwired: 1 in, 4 out]
          }
          frame Enabled {
          }
        }
        n170 = flat-sequence {
          tunnel: w346 -> [w360]
          tunnel: w345 -> [w366]
          frame #0 {
            n171 = call "ExitAllResource.vi"("error in (no error)"=w360) -> ("error out"=w361:errorcluster)  [unwired: 10 in]
            n172 = property class="App"(error in=w361) -> ("App.Kind"=w362:T7)  [unwired: 1 in, 2 out]
            n173 = case shown="\"Run Time System\"" w362 {
              frame "Development System", Default {
              }
              frame "Run Time System" {
                n174 = control-ref of="本VI"() -> (w363:refnum<vi>)
                n175 = invoke class="VI" method="FP.Close"(reference=w363) -> (error out=w364:errorcluster)  [unwired: 2 in, 2 out]
                n176 = call <vilib>:"Clear Errors.vi"("error in (no error)"=w364) -> ()  [unwired: 5 in, 2 out]
              }
            }
          }
          frame #1 {
            n177 = disable-structure shown="禁用" {
              frame Disabled {
                n178 = Quit LabVIEW(quit? (T)=TRUE) -> ()
              }
              frame Enabled {
              }
            }
            n179 = Unbundle By Name(w366) -> ("MainVI"=w365:refnum<vi>)
            n180 = Close Reference(reference=w365) -> ()  [unwired: 1 in, 1 out]
          }
        }
        n181 = call "AMC Destroy Message Queue.vi"("error in (no error)"=w346, "Message Queue in"=w348) -> ("error out"=w347:errorcluster)  [unwired: 9 out]
      }
    }
  }
